vi "AddDatapoint.vi"(3 "error in (no error)":errorcluster, 4 "Sensor info":string[][](array[string]), 5 "Sensor Type":string, 6 "connection reference in":T1) -> (0 "error out":errorcluster, 1 "Temperature":dbl, 2 "connection reference out":T1)   [LabVIEW 2023]
uses:
  <vilib>/addons/database/Connection.llb/Conn ObjectReference.ctl
  <vilib>/addons/database/Connection.llb/Conn Execute.vi
  <vilib>/addons/database/Recordset.llb/Rec Destroy - Connection.vi
  <vilib>/addons/database/NI_Database_API.lvlib
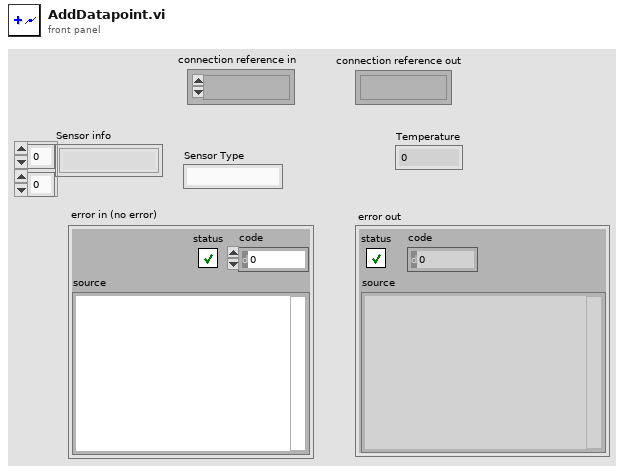
[diagram p1: front panel]
types:
  T1 = typedef "NI_Database_API.lvlib/Conn ObjectReference.ctl" = refnum<k1>
  T2 = typedef "NI_Database_API.lvlib/Rec ObjectReference.ctl" = refnum<k1>
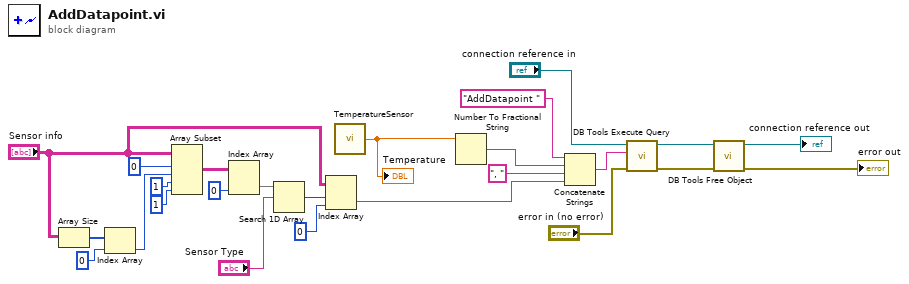
[diagram p0: block diagram]
diagram:
  n1 = Array Size(array="Sensor info") -> (size(s)=w11:i32[])
  n2 = Index Array(array=w11, index=0) -> (element=w2:i32)
  n3 = Array Subset(array="Sensor info", index (row)=0 ("index"), length (row)=w2, index (col)=1 ("index"), length (col)=1 ("length")) -> (w3:string[][])
  n4 = Index Array(array=w3, index (col)=0 ("dimension size")) -> (element=w4:string[])  [unwired: 1 in]
  n5 = Search 1D Array(1D array=w4, element="Sensor Type") -> (index of element=w5:i32)  [unwired: 1 in]
  n6 = Index Array(array="Sensor info", index (row)=w5, index (col)=0 ("index")) -> (element=w1:string)
  n7 = call "TemperatureSensor.vi"() -> ("Temperature"=w15:dbl)  [unwired: 1 in]
  "Temperature" <- w15
  n8 = Number To Fractional String(number=w15) -> (F-format string=w23:string)  [unwired: 3 in]
  n9 = Concatenate Strings("AddDatapoint " ("string"), w23, ", " ("string"), w1) -> (w22:string)
  n10 = call-poly <vilib>:"DB Tools Execute Query.vi"("error in (no error)"="error in (no error)", "SQL query"=w22, "connection reference"="connection reference in") -> ("error out"=w25:errorcluster, "recordset reference"=w24:T2)  [unwired: 5 in]
  n11 = call-poly <vilib>:"DB Tools Free Object.vi"("error in (no error)"=w25, "recordset reference"=w24) -> ("error out"=→"error out":errorcluster, "connection reference"=→"connection reference out":T1)  [unwired: 8 in]
